vi "10.2 Writing DAQmx Data to a File.vi"() -> ()   [LabVIEW 2019]
uses:
  <vilib>/DAQmx/read.llb/DAQmx Read (Analog DBL 1Chan 1Samp).vi
  <vilib>/DAQmx/create/channels.llb/DAQmx Create Channel (AI-Temperature-Thermocouple).vi
  <vilib>/DAQmx/configure/timing.llb/DAQmx Timing (Sample Clock).vi
  <vilib>/DAQmx/miscellaneous.llb/DAQmx Fill In Error Info.vi
panel:
  in  "Configuration Control":T1={"number of samples"=-1, "Minimum Value"=-1.0, "Maximum Value"=-1.0, "physical channels"="Multi_I-O/ai0", "Desired Sample Rate (Hz)"=-1.0, "sample mode"=10178} {"sample mode" items=["Finite Samples"=10178, "Continuous Samples"=10123, "Hardware Timed Single Point"=12522]}
  out "Waveform Chart":dbl(graph)
  in  "File Path Control":path
  in  "Stop":bool
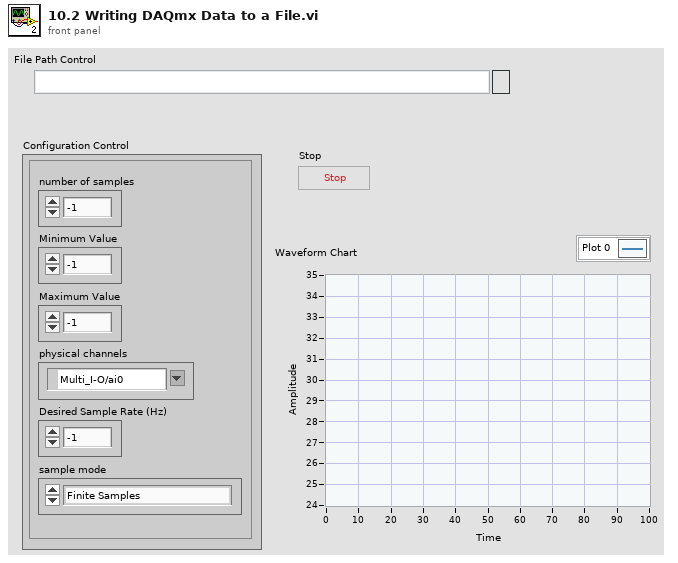
[diagram p1: front panel]
types:
  T1 = cluster{"number of samples":i32, "Minimum Value":dbl, "Maximum Value":dbl, "physical channels":tag, "Desired Sample Rate (Hz)":dbl, "sample mode":i32}
  T2 = enum16{"open", "replace", "create", "open or create", "replace or create", "replace or create with confirmation"}
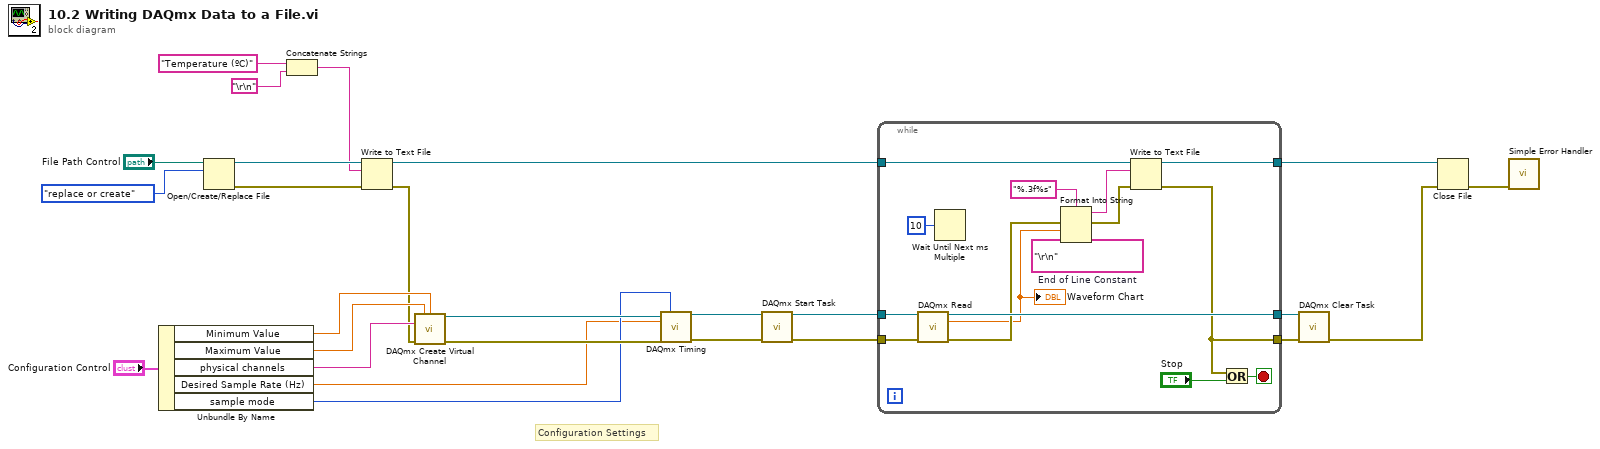
[diagram p0: block diagram]
diagram:
  # "Configuration Settings"
  n1 = Unbundle By Name("Configuration Control") -> ("Minimum Value"=w7:dbl, "Maximum Value"=w8:dbl, "physical channels"=w6:tag, "Desired Sample Rate (Hz)"=w4:dbl, "sample mode"=w5:i32)
  n2 = Open/Create/Replace File(file path (use dialog)="File Path Control", operation (0:open)=T2."replace or create") -> (refnum out=w20:refnum<file>, error out=w19:errorcluster)  [unwired: 4 in, 1 out]
  n3 = Concatenate Strings "Concatenate Strings"("Temperature (ºC)", "\r\n") -> (w16:string)
  n4 = Write to Text File(file (use dialog)=w20, text=w16, error in=w19) -> (refnum out=w15:refnum<file>, error out=w2:errorcluster)  [unwired: 1 in, 1 out]
  n5 = call-poly <vilib>:"DAQmx Create Virtual Channel.vi"("maximum value"=w8, "minimum value"=w7, "physical channels"=w6, "error in"=w2) -> ("task out"=w11:refnum<k21>, "error out"=w10:errorcluster)  [unwired: 10 in]
  n6 = call-poly <vilib>:"DAQmx Timing.vi"("task/channels in"=w11, "sample mode"=w5, "rate"=w4, "error in"=w10) -> ("task out"=w1:refnum<k21>, "error out"=w3:errorcluster)  [unwired: 10 in]
  n7 = call <vilib>:"DAQmx Start Task.vi"("task/channels in"=w1, "error in"=w3) -> ("task out"=w26:refnum<k21>, "error out"=w24:errorcluster)  [unwired: 12 in]
  n8 = while {
    tunnel: w26 -> [w41]
    tunnel: [w40] -> w25
    tunnel: w24 -> [w39]
    tunnel: [w31] -> w23
    tunnel: w15 -> [w33]
    tunnel: [w30] -> w14
    stop <- w36 stop-if-true
    w37 = "\r\n"  # End of Line Constant
    n9 = call-poly <vilib>:"DAQmx Read.vi"("task/channels in"=w41, "error in"=w39) -> ("task out"=w40:refnum<k21>, "data"=w27:dbl, "error out"=w34:errorcluster)  [unwired: 11 in]
    "Waveform Chart" <- w27
    n10 = Wait Until Next ms Multiple(millisecond multiple=u32 10) -> ()  [unwired: 1 out]
    n11 = Format Into String(format string="%.3f%s", error in=w34, w27, w37) -> (resulting string=w29:string, error out=w32:errorcluster)  [unwired: 1 in]
    n12 = Write to Text File(file (use dialog)=w33, text=w29, error in=w32) -> (refnum out=w30:refnum<file>, error out=w31:errorcluster)  [unwired: 1 in, 1 out]
    n13 = Or(x=w31, y="Stop") -> (x .or. y?=w36:bool)
  }
  n14 = call <vilib>:"DAQmx Clear Task.vi"("task in"=w25, "error in"=w23) -> ("error out"=w13:errorcluster)  [unwired: 13 in]
  n15 = Close File(refnum=w14, error in=w13) -> (error out=w12:errorcluster)  [unwired: 1 out]
  n16 = call <vilib>:"Simple Error Handler.vi"("error in (no error)"=w12) -> ()  [unwired: 4 in, 5 out]
